vi "KM101_RotateNegtive.vi"(9 "Channel":i32, 10 "reference in":refnum<k7>) -> (1 "Steps":i32, 2 "reference out":refnum<k7>)   [LabVIEW 2018, in "KIM101lib.lvlib"]
uses:
  KIM101lib.lvlib
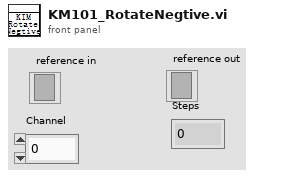
[diagram p1: front panel]
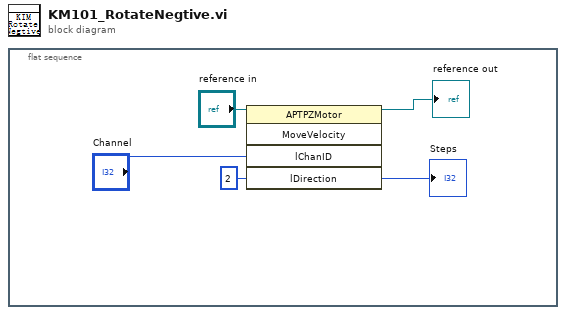
[diagram p0: block diagram]
diagram:
  n1 = flat-sequence {
    frame #0 {
      n2 = invoke class="APTPZMotor" method="MoveVelocity"(reference="reference in", "lChanID"="Channel", "lDirection"=2) -> (reference out=→"reference out":refnum<k7>, "lDirection"=→"Steps":i32)  [unwired: 2 in, 3 out]
    }
  }
